vi "Save Panel.vi"(8 "error in (no error)":errorcluster, 10 "vi reference":refnum<vi>) -> (0 "error out":errorcluster, 2 "output cluster":cluster{i32[][], string[]})   [LabVIEW 2015]
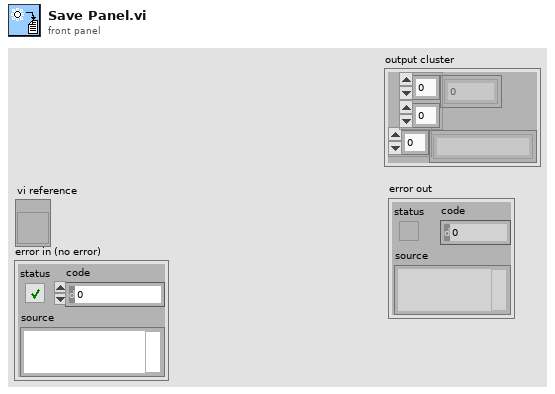
[diagram p1: front panel]
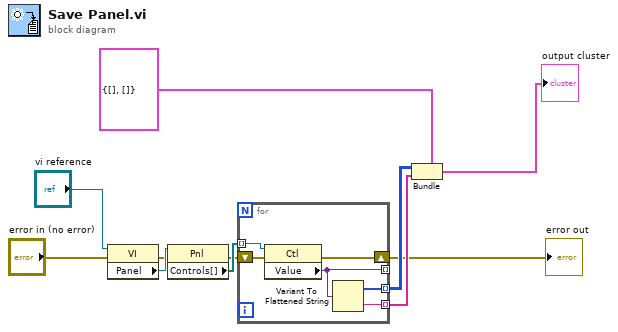
[diagram p0: block diagram]
diagram:
  n1 = property class="VI"(reference="vi reference", error in="error in (no error)") -> (error out=w8:errorcluster, "Panel"=w10:refnum<vi>)  [unwired: 1 out]
  n2 = property class="Pnl"(reference=w10, error in=w8) -> (error out=w6:errorcluster, "Controls[]"=w7:refnum<vi>[])  [unwired: 1 out]
  n3 = for {
    tunnel: [w17] -> _ mode=indexing
    tunnel: [w16] -> w4 mode=indexing
    tunnel: [w15] -> w3 mode=indexing
    tunnel: w7 -> [w14] mode=indexing
    shift-right: [w12] -> w1
    shift-left: w6 -> [w13]
    n4 = property class="Ctl"(reference=w14, error in=w13) -> (error out=w12:errorcluster, "Value"=w17:variant)  [unwired: 1 out]
    n5 = Variant To Flattened String(Variant=w17) -> (data string=w15:string, 1:w16:i16[])
  }
  "error out" <- w1
  n6 = Bundle(cluster=cluster{i32[][], string[]} {[], []} ("input cluster"), w4, w3) -> (→"output cluster":cluster{i32[][], string[]})
